vi "BotSpeak_RIO_LED.vi"(2 "LED":u8(slide)=1 scale=1.0..6.0, 3 "State":bool=TRUE, 4 "Bot Settings":T1) -> (0 "response":string="169.254.32.85", 1 "Bot Settings 2":T1)   [LabVIEW 2012]
doc: "Sets the state of the specified RIO \"LED\" to high or low acording to the boolean \"State\"."
uses:
  <userlib>/BotSpeak/VIs/Direct/BotSpeak_Control.ctl
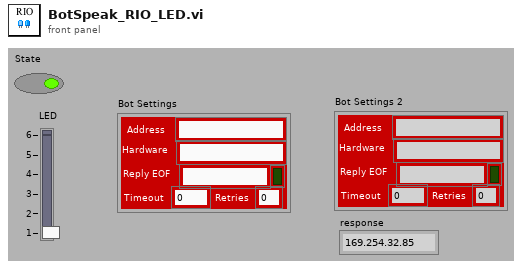
[diagram p1: front panel]
types:
  T1 = typedef "BotSpeak_Control.ctl" = cluster{"Address":string, "Reply EOF":string, "Hardware":string, "Retries":i8, "Timeout":i32, "Open?":bool}
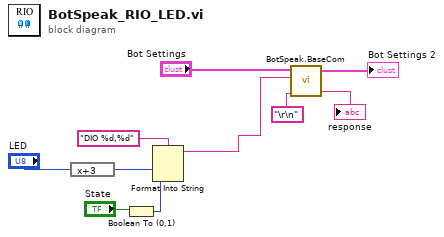
[diagram p0: block diagram]
diagram:
  n1 = expression code="x+3"("LED") -> (w6:u8)
  n2 = Boolean To (0,1)(Boolean="State") -> (0, 1=w7:i16)
  n3 = Format Into String(format string="DIO %d,%d" ("command"), w6, w7) -> (resulting string=w1:string)  [unwired: 2 in, 1 out]
  n4 = call <userlib>:"BotSpeak.BaseCom.vi"("Termination"="\r\n", "command"=w1, "Bot Settings in"="Bot Settings") -> ("response"=→"response":string, "Bot Settings out"=→"Bot Settings 2":T1)  [unwired: 2 in]
